vi "_Test - Get Control Pos Info.vi"() -> ()   [LabVIEW 2024, in "EQMF.lvlib" / "Controls.lvlib"]
uses:
  Controls.lvlib
panel:
  in  "Parent Tab Pos":T1(ring)
  in  "Child Tab Pos":T1(ring)
  in  "dY":i32
  in  "dX":i32
  in  "Tab Control":enum32{"Page 1", "Page 2"}(tab)
  in  "Tab Control 2":enum32{"Page 1", "Page 2"}(tab)
  in  "OK Button 2":bool
  in  "OK Button":bool
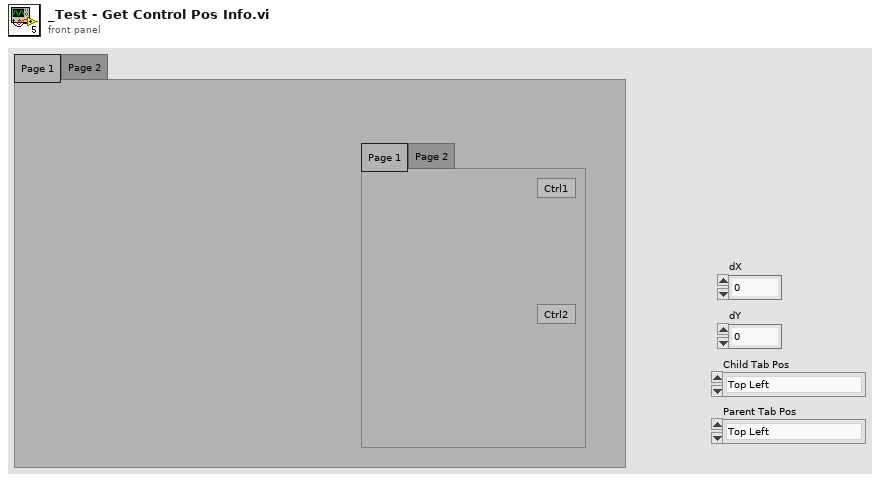
[diagram p1: front panel]
types:
  T1 = enum16{"Top Left", "Top Right", "Bottom Left", "Bottom Right"}
  T2 = enum16{"Top Left", "Top Right", "Bottom Left", "Bottom Right", "Left", "Right", "Top", "Bottom"}
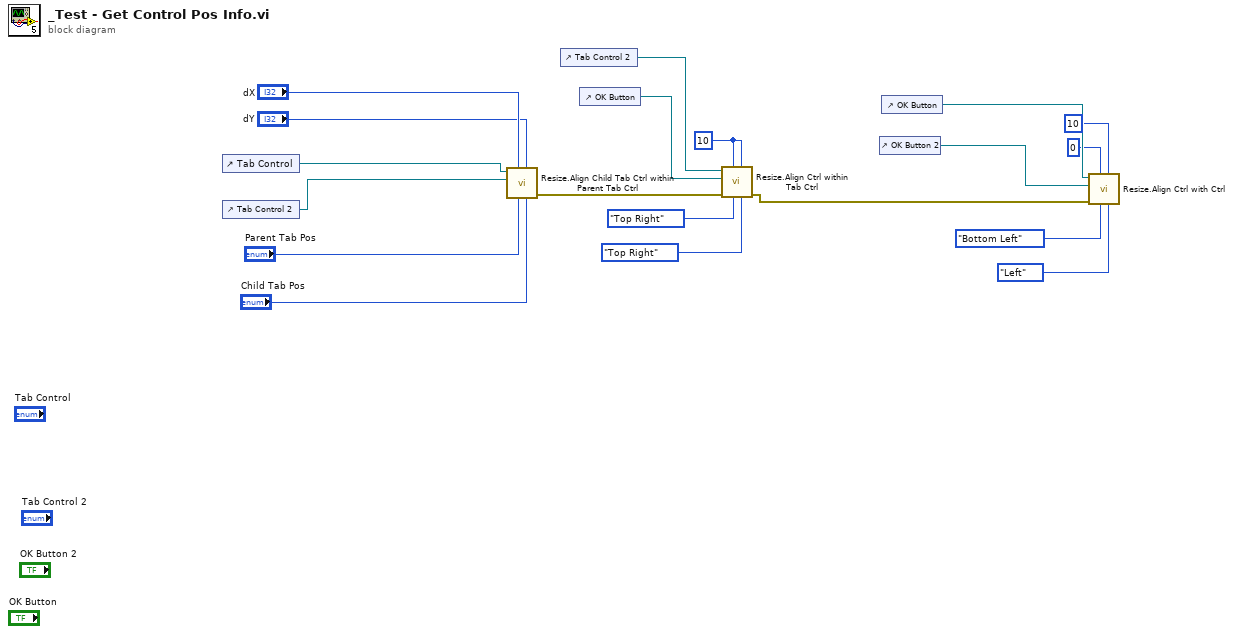
[diagram p0: block diagram]
diagram:
  w3 = 10 ("dX")
  n1 = control-ref of="Tab Control"() -> (w17:refnum<vi>)
  n2 = control-ref of="Tab Control 2"() -> (w16:refnum<vi>)
  n3 = call "Resize.Align Child Tab Ctrl within Parent Tab Ctrl.vi"("Child Ref Pos"="Child Tab Pos", "dY"="dY", "Parent Ref Pos"="Parent Tab Pos", "dX"="dX", "Child Tab Ctrl"=w16, "Parent Tab Ctrl"=w17) -> ("error out"=w5:errorcluster)  [unwired: 3 in, 2 out]
  n4 = control-ref of="Tab Control 2"() -> (w6:refnum<vi>)
  n5 = control-ref of="OK Button"() -> (w7:refnum<vi>)
  n6 = call "Resize.Align Ctrl within Tab Ctrl.vi"("Child Ref Pos"=T1."Top Right", "dY"=w3, "Parent Ref Pos"=T1."Top Right", "dX"=w3, "error in"=w5, "Child Ctrl"=w7, "Parent Tab Ctrl"=w6) -> ("error out"=w4:errorcluster)  [unwired: 2 in, 2 out]
  n7 = control-ref of="OK Button 2"() -> (w12:refnum<vi>)
  n8 = control-ref of="OK Button"() -> (w13:refnum<vi>)
  n9 = call "Resize.Align Ctrl with Ctrl.vi"("Move Ctrl Ref Location"=T2."Left", "dY"=10, "Ref Ctrl Corner"=T1."Bottom Left", "dX"=0, "error in"=w4, "Move Ctrl"=w12, "Ref Ctrl"=w13) -> ()  [unwired: 2 in, 3 out]
